vi "A_Graph Sub.vi"(0 "Set Point Shift":dbl[](array[numeric]), 1 "New Set Pt":dbl, 2 "Ramp Rate Shift":dbl[](array[numeric]), 3 "Time Shift":dbl[](array[numeric]), 4 "New Time":dbl, 5 "New Error":dbl, 6 "New Ramp Rate":dbl[](array[numeric]) format="%0.2f", 7 "Error Shift":dbl[](array[numeric]), 8 "New Actual":dbl, 10 "Actual Shift":dbl[](array[numeric]), 13 "New Vial":dbl, 19 "Vial Shift":dbl[](array[numeric])) -> (11 "Vial Out":dbl[](array[numeric]), 12 "Actual Out":dbl[](array[numeric]), 14 "Graph Out":cluster{dbl[], dbl[]}[](array[cluster]), 15 "Set Pt Out":dbl[](array[numeric]), 16 "Ramp Rate Out":dbl[](array[numeric]), 17 "Time Out":dbl[](array[numeric]), 18 "Error Out":dbl[](array[numeric]))   [LabVIEW 2011]
uses:
  <vilib>/Analysis/NI_AALBase.lvlib
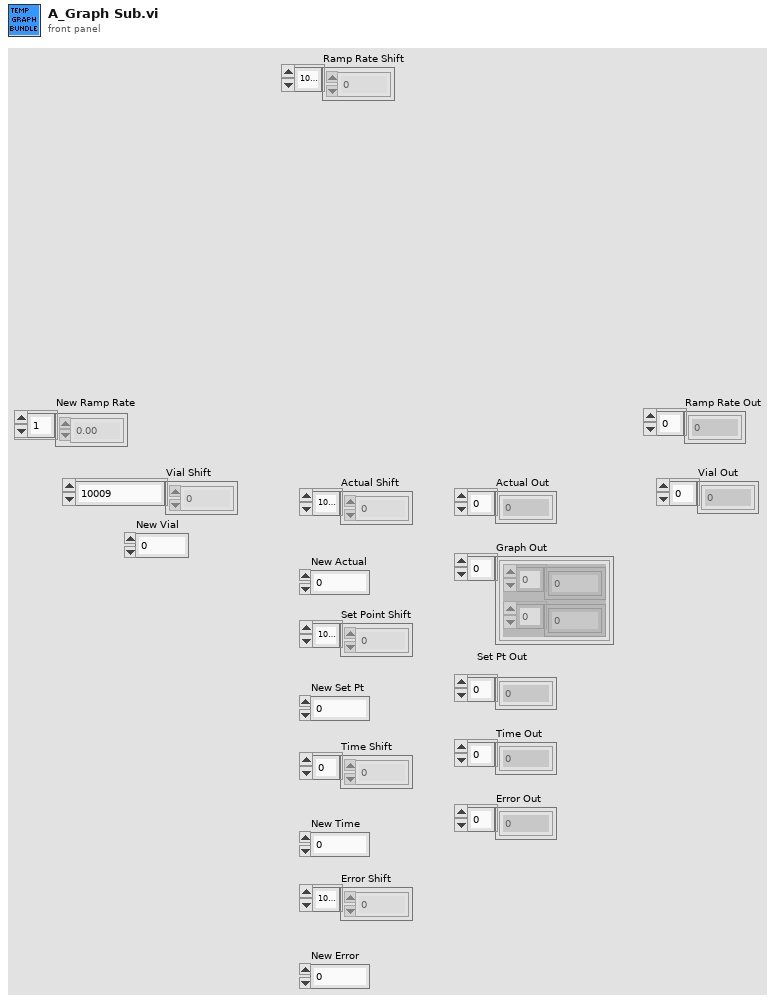
[diagram p1: front panel]
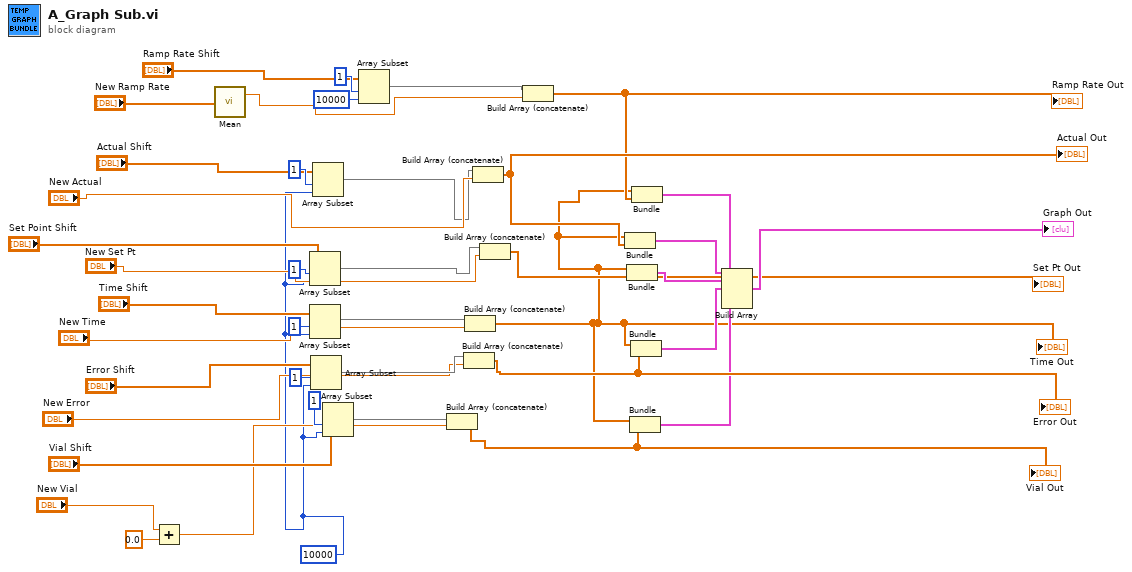
[diagram p0: block diagram]
diagram:
  w10 = 10000 ("length")
  n1 = Add(x="New Vial", y=0.0) -> (x+y=w14:dbl)
  n2 = call <vilib>:"Mean.vi"("X"="New Ramp Rate") -> ("mean"=w6:dbl)  [unwired: 1 out]
  n3 = Array Subset(array="Set Point Shift", index=1, length=w10) -> (w28:dbl[])
  n4 = Array Subset(array="Time Shift", index=1, length=w10) -> (w34:dbl[])
  n5 = Array Subset(array="Error Shift", index=1, length=w10) -> (w30:dbl[])
  n6 = Array Subset(array="Actual Shift", index=1, length=w10) -> (w5:dbl[])
  n7 = Array Subset(array="Vial Shift", index=1, length=w10) -> (w18:dbl[])
  n8 = Array Subset(array="Ramp Rate Shift", index=1, length=10000) -> (w2:dbl[])
  n9 = Build Array (concatenate)(w18, w14) -> (w17:dbl[])
  "Vial Out" <- w17
  n10 = Build Array (concatenate)(w30, "New Error") -> (w29:dbl[])
  "Error Out" <- w29
  n11 = Build Array (concatenate)(w34, "New Time") -> (w7:dbl[])
  "Time Out" <- w7
  n12 = Build Array (concatenate)(w5, "New Actual") -> (w26:dbl[])
  "Actual Out" <- w26
  n13 = Build Array (concatenate)(w28, "New Set Pt") -> (w27:dbl[])
  "Set Pt Out" <- w27
  n14 = Build Array (concatenate)(w2, w6) -> (w8:dbl[])
  "Ramp Rate Out" <- w8
  n15 = Bundle(w7, w26) -> (w39:cluster{dbl[], dbl[]})  [unwired: 1 in]
  n16 = Bundle(w7, w27) -> (w38:cluster{dbl[], dbl[]})  [unwired: 1 in]
  n17 = Bundle(w7, w17) -> (w16:cluster{dbl[], dbl[]})  [unwired: 1 in]
  n18 = Bundle(w7, w29) -> (w37:cluster{dbl[], dbl[]})  [unwired: 1 in]
  n19 = Bundle(w7, w8) -> (w1:cluster{dbl[], dbl[]})  [unwired: 1 in]
  n20 = Build Array(w39, w38, w37, w16, w1) -> (→"Graph Out":cluster{dbl[], dbl[]}[])
